vi "wrap.RunString.vi"(0 "class.GLue in":refnum<class "class.GLue.lvclass">, 2 "Script":string, 11 "error in (no error)":errorcluster) -> (4 "class.GLue out":refnum<class "class.GLue.lvclass">, 12 "return type":i32, 14 "Error":string, 15 "error out":errorcluster)   [LabVIEW 2014, in "GLue.lvlib" / "class.GLue.lvclass"]
uses:
  class.GLue.lvclass
  class.GLue.lvclass/class.GLue.ctl
  Resources/GLue.dll
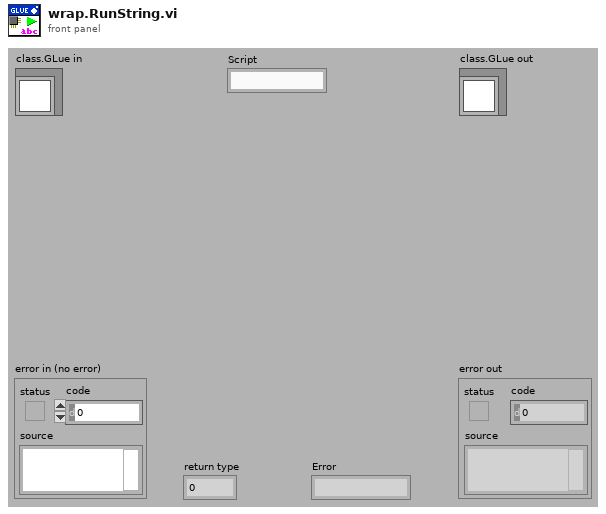
[diagram p1: front panel]
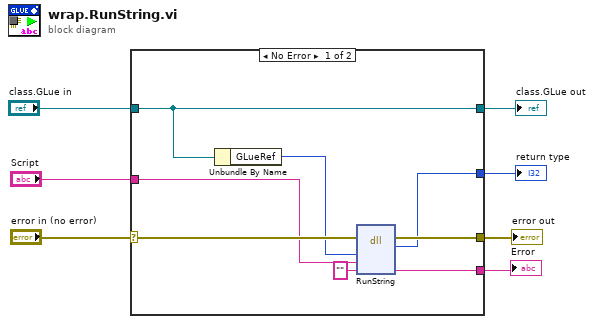
[diagram p0: block diagram]
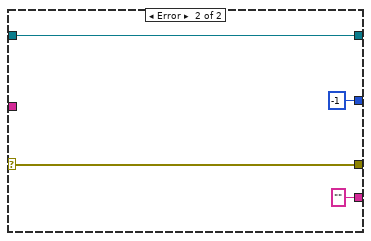
[diagram p2: hidden frame]
diagram:
  n1 = case shown="No Error" "error in (no error)" {
    selector: "error in (no error)" -> [w14 w19]
    tunnel: [w13 w19] -> w6
    tunnel: [w15 w18] -> w4
    tunnel: "class.GLue in" -> [w15 w18]
    tunnel: "Script" -> [w11 _]
    tunnel: [w9 -1 ("return type")] -> w2
    tunnel: [w8 "" ("Error")] -> w1
    frame No Error {
      n2 = Unbundle By Name(w15) -> ("GLueRef"=w12:i64)
      n3 = dll-call lib="C:/Users/Antonie/Documents/work/glue/trunk/Resources/GLue.dll" fn="RunString"(error in=w14, "GLue"=w12, "Script"=w11, "Error"="") -> (error out=w13:errorcluster, "return type"=w9:i32, "Error"=w8:string)  [unwired: 4 in, 1 out]
    }
    frame Error {
    }
  }
  "error out" <- w6
  "class.GLue out" <- w4
  "return type" <- w2
  "Error" <- w1
